vi "FGV - Acquisition Status.vi"(5 "mem loc":i32, 7 "Actions":T2=enum."Clear", 8 "Error In":errorcluster, 9 "Quit status":bool, 10 "Scan Type [In]":T1, 11 "Level Status In":bool) -> (0 "Error Out":errorcluster, 1 "Quit status out":bool, 2 "Scan Type [Out]":T1, 3 "Level Status out":bool, 4 "mem loc out":i32)   [LabVIEW 2018]
uses:
  Controls/FGV Actions.ctl
  Controls/ScanType.ctl
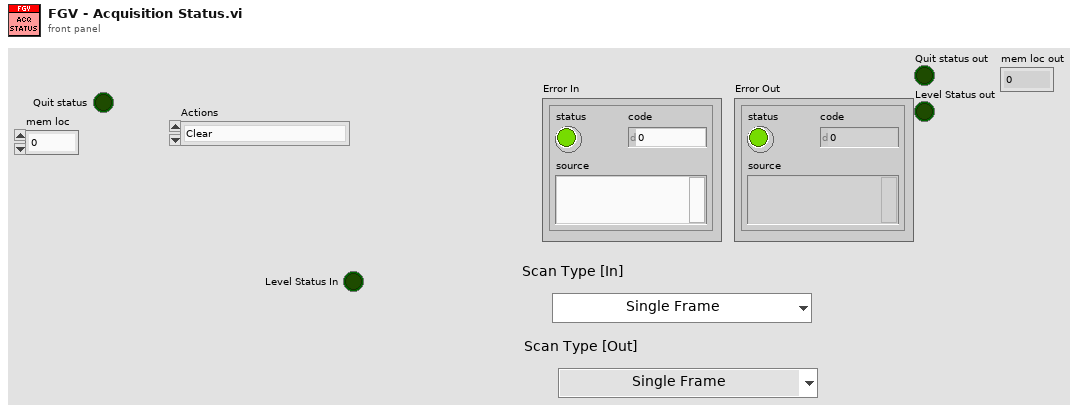
[diagram p1: front panel]
types:
  T1 = typedef "ScanType.ctl" = enum16{"Single Frame", "Continuous Frame", "ROI Line", "Vibratome", "Mosaic", "Mosaic + Slice"}
  T2 = typedef "FGV Actions.ctl" = enum16{"Init", "Set", "Get", "Clear"}
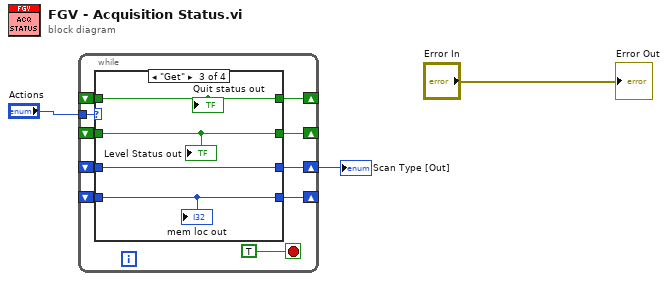
[diagram p0: block diagram]
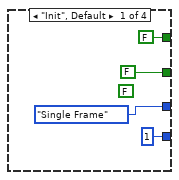
[diagram p2: hidden frame]
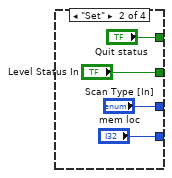
[diagram p3: hidden frame]
diagram:
  n1 = while {
    tunnel: "Actions" -> [w12]
    shift-right: [w11] -> w1
    shift-left: _ -> [w10]
    shift-right: [w9] -> _
    shift-left: _ -> [w8]
    shift-right: [w7] -> _
    shift-left: _ -> [w6]
    shift-right: [w5] -> _
    shift-left: _ -> [w4]
    stop <- TRUE stop-if-true
    n2 = case shown="\"Get\"" w12 {
      tunnel: [ScanType."Single Frame" ("Scan Type") "Scan Type [In]" w25 _] -> w11
      tunnel: w10 -> [_ _ w25 _]
      tunnel: [FALSE ("Quit status") "Quit status" w24 _] -> w9
      tunnel: w8 -> [_ _ w24 _]
      tunnel: [FALSE "Level Status In" w23 _] -> w7
      tunnel: w6 -> [_ _ w23 _]
      tunnel: [1 ("mem loc") "mem loc" w22 _] -> w5
      tunnel: w4 -> [_ _ w22 _]
      frame "Init", Default {
        (unwired) FALSE
      }
      frame "Set" {
      }
      frame "Get" {
        "Quit status out" <- w24
        "Level Status out" <- w23
        "mem loc out" <- w22
      }
      frame "Clear" {
      }
    }
  }
  "Scan Type [Out]" <- w1
  "Error Out" <- "Error In"
